vi "Test Process Restarting Maintains State.vi"(8 "error in (no error)":errorcluster, 11 "Process Test In":refnum<class "Process Dev Test.lvclass">) -> (0 "error out":errorcluster, 3 "Process Test Out":refnum<class "Process Dev Test.lvclass">)   [LabVIEW 2020, in "Process Dev Test.lvclass"]
uses:
  Process Dev Test.lvclass
  C:/Program Files (x86)/National Instruments/LabVIEW 2020/vi.lib/Astemes/LUnit/Test Case.lvclass
  source/Framework/Process/Process.lvclass/Process.ctl
  <vilib>/Astemes/LUnit/Test Case.lvclass/Test Case.ctl
  <vilib>/Astemes/LUnit/LUnit Assertion Result.lvclass/LUnit Assertion Result.ctl
  <vilib>/Astemes/LUnit/LUnit Test Case Result.lvclass/LUnit Test Case Result.ctl
  <vilib>/Astemes/LUnit/LUnit Method Result.lvclass/LUnit Method Result.ctl
  source/Framework/Process/Private/SubVIs/Wait for finish.vi
  source/Framework/Process/Protected/Messaging/Enqueue Message.vi
  source/Framework/Process/Private/SubVIs/Set Lifecycle State.vi
  source/Framework/Process/Public/Lifecycle/Get Lifecycle State.vi
  <vilib>/Astemes/LUnit/Palette/Fail.vi
  <vilib>/Astemes/LUnit/Palette/Pass.vi
  <vilib>/Astemes/LUnit/Set Assertion Type.vi
  source/Framework/Process/Private/SubVIs/Handle Debug Data.vi
  <vilib>/Utility/error.llb/Clear Errors.vi
  <vilib>/Astemes/LUnit/Add test result.vi
  <vilib>/Astemes/LUnit/LUnit Write Passed.vi
  <vilib>/Astemes/LUnit/LUnit Write Message.vi
  <vilib>/Astemes/LUnit/LUnit Write Description.vi
  <vilib>/Astemes/LUnit/LUnit Write Assertion Type.vi
  source/Framework/Logging/Log Debug.vi
  <vilib>/AdvancedString/1D String Array to Delimited String.vi
  <vilib>/Utility/High Resolution Relative Seconds.vi
  <vilib>/Astemes/LUnit/LUnit Record Assertion Result.vi
  <vilib>/Astemes/LUnit/LUnit Aggregate Assertion Results.vi
  <vilib>/Astemes/LUnit/Assertion Result/LUnit Read Status.vi
  <vilib>/Astemes/LUnit/LUnit Read Message.vi
  <vilib>/Astemes/LUnit/LUnit Read Description.vi
  <vilib>/Astemes/LUnit/Method Result/LUnit Merge Status.vi
  <vilib>/Astemes/LUnit/LUnit Concatenate result strings.vi
  <vilib>/Utility/error.llb/Error Cluster From Error Code.vi
  source/Framework/Process/Public/Read Name.vi
  <vilib>/Astemes/LUnit/LUnit Assertion Result.lvclass
  source/Framework/Process/Process.lvclass
  Process Dev Test.lvclass/Process Dev Test.ctl
  <vilib>/Astemes/LUnit/Test Case.lvclass
  97bcfca7-9139-4f20-8796-160450356e69.vi
  C:/Git/astemes-triarc-framework/source/Framework Test Suite/Base Class Test/Base Test.lvclass
  C:/Git/astemes-triarc-framework/tests/Process Development Test/Process Test/Process Dev Test.lvclass
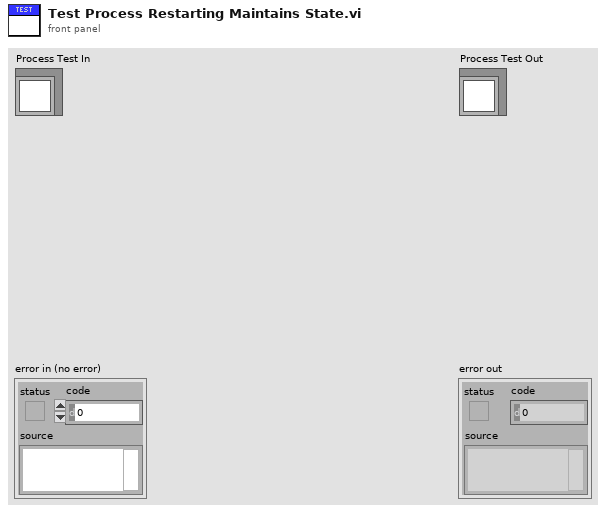
[diagram p1: front panel]
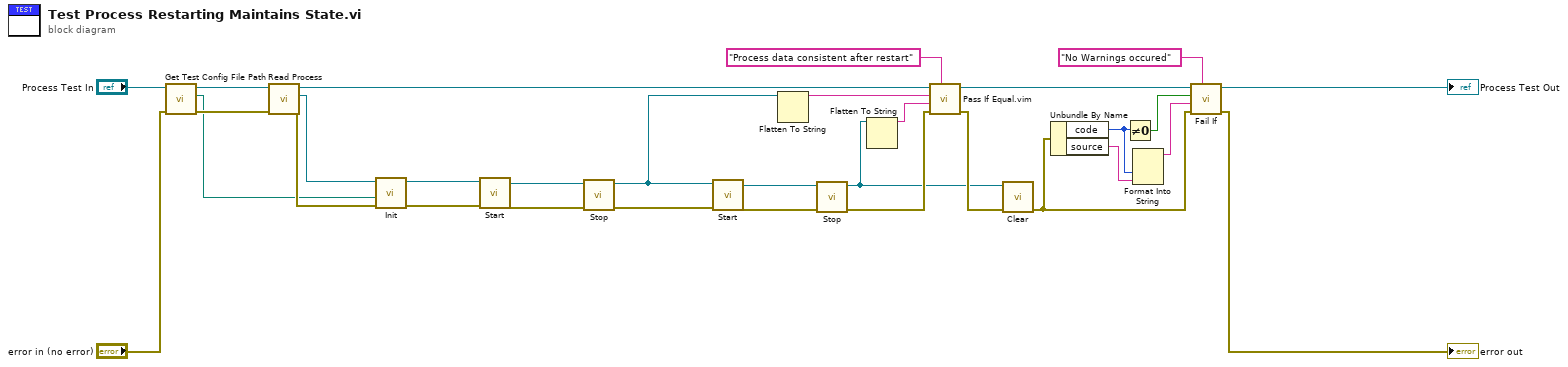
[diagram p0: block diagram]
diagram:
  n1 = call "Get Test Config File Path.vi"("error in (no error)"="error in (no error)", "Process Test In"="Process Test In") -> ("error out"=w22:errorcluster, "Test config path"=w5:path, "Process Test Out"=w26:refnum<class "Process Dev Test.lvclass">)  [unwired: 7 in]
  n2 = call "Read Process.vi"("error in (no error)"=w22, "Process Test in"=w26) -> ("error out"=w23:errorcluster, "Process.lvclass"=w6:refnum<class "Process.lvclass">, "Process Test out"=w24:refnum<class "Process Dev Test.lvclass">)  [unwired: 7 in]
  n3 = call-dynamic "Init.vi"("error in (no error)"=w23, "Config File Path"=w5, "Process In"=w6) -> ("error out"=w27:errorcluster, "Process Out"=w28:refnum<class "Process.lvclass">)  [unwired: 7 in]
  n4 = call "Start.vi"("error in (no error)"=w27, "Process In"=w28) -> ("error out"=w30:errorcluster, "Process Out"=w31:refnum<class "Process.lvclass">)  [unwired: 7 in, 1 out]
  n5 = call "Stop.vi"("error in (no error)"=w30, "Process In"=w31) -> ("error out"=w7:errorcluster, "Process Out"=w4:refnum<class "Process.lvclass">)  [unwired: 7 in, 1 out]
  n6 = call "Start.vi"("error in (no error)"=w7, "Process In"=w4) -> ("error out"=w13:errorcluster, "Process Out"=w12:refnum<class "Process.lvclass">)  [unwired: 7 in, 1 out]
  n7 = Flatten To String(anything=w4) -> (data string=w1:string)  [unwired: 3 in, 2 out]
  n8 = call "Stop.vi"("error in (no error)"=w13, "Process In"=w12) -> ("error out"=w10:errorcluster, "Process Out"=w3:refnum<class "Process.lvclass">)  [unwired: 7 in, 1 out]
  n9 = Flatten To String(anything=w3) -> (data string=w2:string)  [unwired: 3 in, 2 out]
  n10 = call "Pass If Equal.vim"("Description"="Process data consistent after restart", "error in (no error)"=w10, "Actual"=w2, "Expected"=w1, "LUnit Test Case In"=w24) -> ("error out"=w9:errorcluster, "LUnit Test Case Out"=w11:refnum<class "Process Dev Test.lvclass">)  [unwired: 5 in]
  n11 = call-dynamic "Clear.vi"("error in (no error)"=w9, "Process In"=w3) -> ("error out"=w18:errorcluster)  [unwired: 9 in]
  n12 = Unbundle By Name(w18) -> ("code"=w16:i32, "source"=w14:string)
  n13 = Not Equal To 0?(x=w16) -> (x != 0?=w20:bool)
  n14 = Format Into String(w16, w14) -> (resulting string=w15:string)  [unwired: 3 in, 1 out]
  n15 = call <vilib>:"Fail If.vi"("Description"="No Warnings occured", "error in (no error)"=w18, "Message"=w15, "Fail?"=w20, "LUnit Test Case In"=w11) -> ("error out"=→"error out":errorcluster, "LUnit Test Case Out"=→"Process Test Out":refnum<class "Process Dev Test.lvclass">)  [unwired: 5 in]
